vi "Timing.Get Priority.vi"(11 "Timing in":refnum<class "Timing.lvclass">) -> (2 "Priority":u64, 3 "Timing out":refnum<class "Timing.lvclass">)   [LabVIEW 2017, in "DSF Core.lvlib" / "Timing.lvclass"]
uses:
  Timing.lvclass
  Timing.lvclass/Timing.ctl
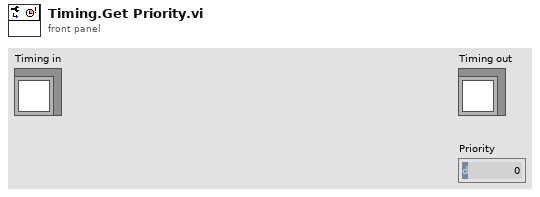
[diagram p1: front panel]
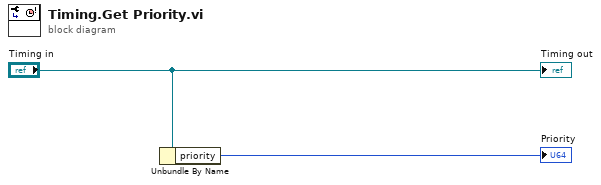
[diagram p0: block diagram]
diagram:
  n1 = Unbundle By Name("Timing in") -> ("priority"=→"Priority":u64)
  "Timing out" <- "Timing in"
